vi "Save Recording.vi"(8 "error in":errorcluster, 9 "Save":bool, 11 "Interface In":T1) -> (0 "error out":errorcluster, 1 "Save?":bool, 2 "Data":fxp<+/-,8,8>[](array[numeric]), 3 "Interface Out":T1)   [LabVIEW 2015]
uses:
  TypeDefs Host/FPGA Dynamic Interface.ctl
  TypeDefs Host/Open Audio FGV Enum.ctl
  <vilib>/Utility/error.llb/Error Cluster From Error Code.vi
  <vilib>/rvi/errors/niLvFpgaAdjustHostInterfaceError.vi
  <vilib>/rvi/interface/common/niFpgaWaitOnOcc.vi
  <vilib>/rvi/interface/nirviReadWriteControl/nirviReadWriteControl.xnode
  <vilib>/rvi/interface/nirviMethod/nirviMethod.xnode
  <vilib>/rvi/errors/niLvFpgaMergeErrorWithErrorCode.vi
  <vilib>/FPGAPlugInAG/Dynamic/niLvFpga_ReadFifo_Dynamic.vi
  NiFpgaLv.dll
  <vilib>/rvi/interface/Simulation/niFpgaSimulationCallBeginRW.vi
  <vilib>/FPGAPlugInAG/Dynamic/niLvFpga_ConfigureFifo_Dynamic.vi
  <vilib>/FPGAPlugInAG/Dynamic/niLvFpga_StartFifo_Dynamic.vi
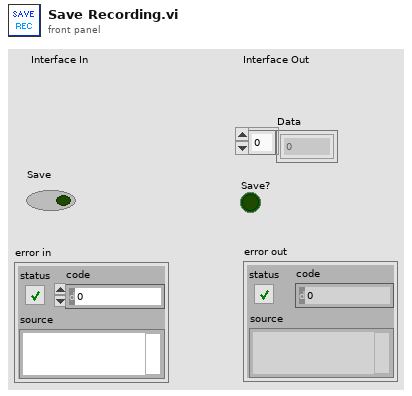
[diagram p1: front panel]
types:
  T1 = typedef "FPGA Dynamic Interface.ctl" = refnum<k20>
  T2 = typedef "Open Audio FGV Enum.ctl" = enum16{"Get", "Set"}
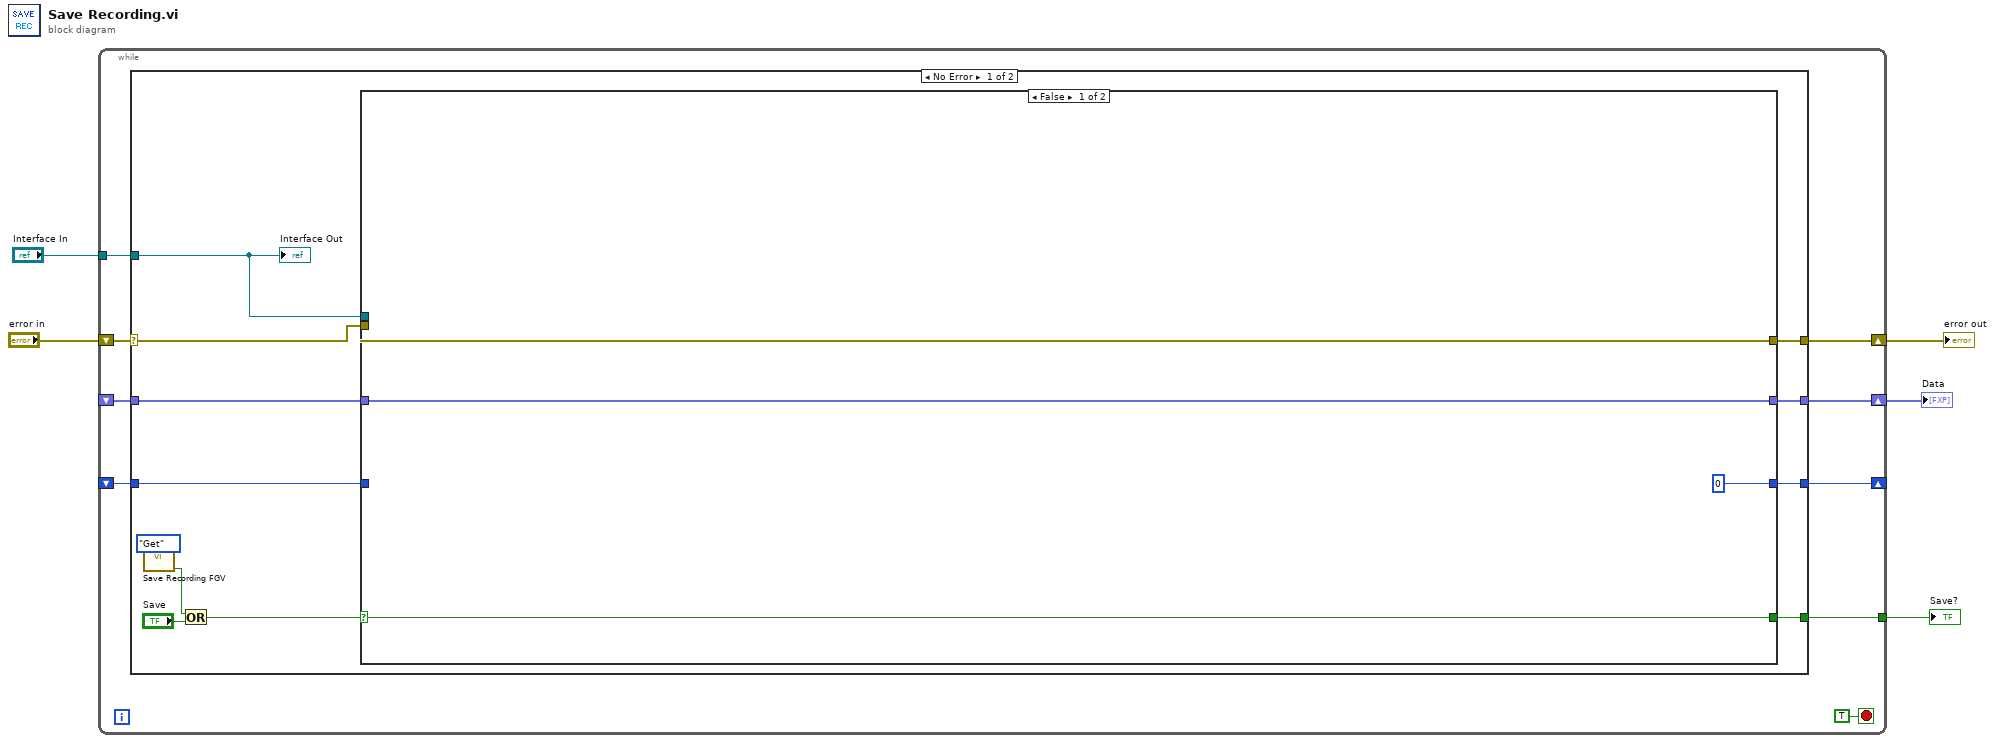
[diagram p0: block diagram]
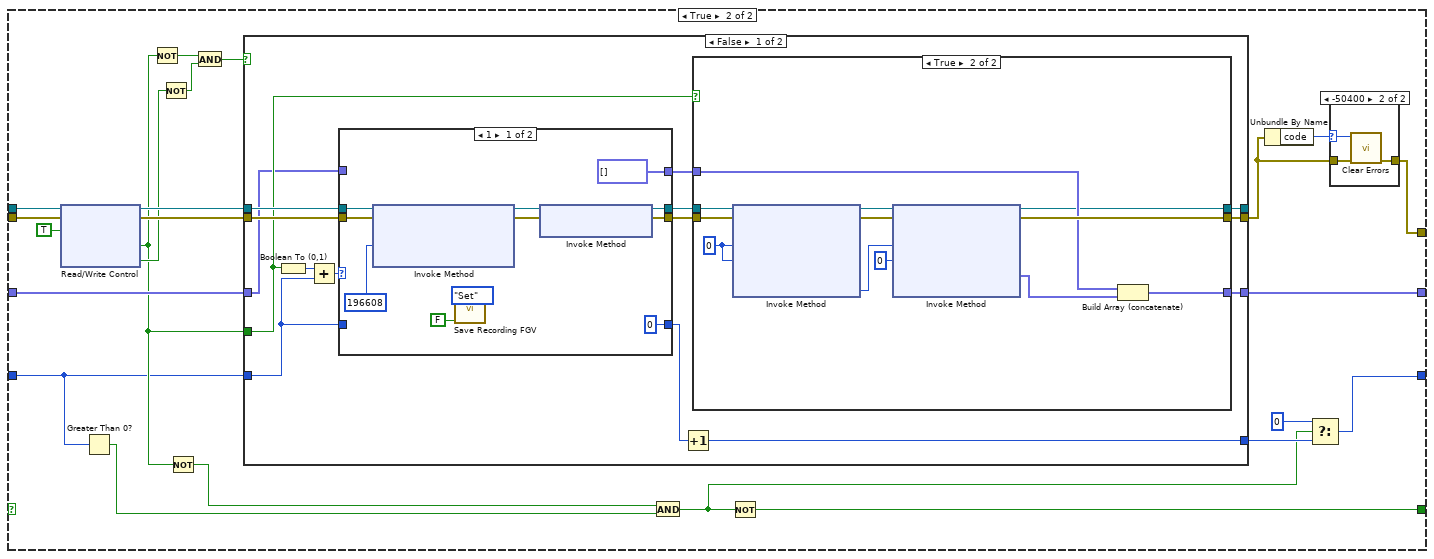
[diagram p2: hidden frame]
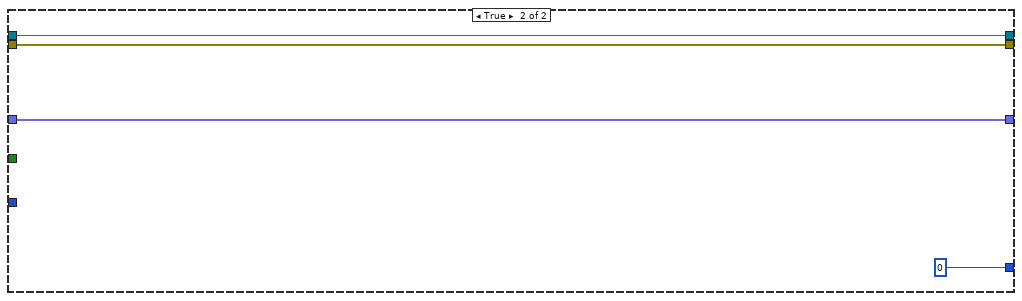
[diagram p6: hidden frame]
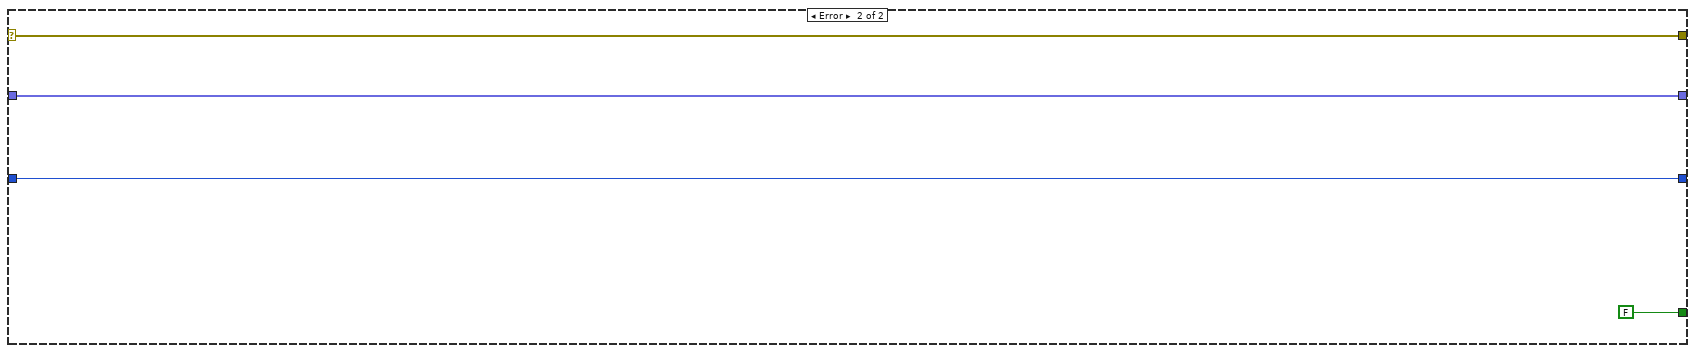
[diagram p7: hidden frame]
diagram:
  n1 = while {
    shift-right: [w10] -> w2
    shift-left: "error in" -> [w7]
    shift-right: [w14] -> w4
    shift-left: _ -> [w12]
    shift-right: [w11] -> _
    shift-left: _ -> [w13]
    tunnel: [w8] -> w3
    tunnel: "Interface In" -> [w6]
    stop <- TRUE stop-if-true
    n2 = case shown="No Error" w7 {
      selector: w7 -> [w16 w110]
      tunnel: [w26 w109] -> w14
      tunnel: w13 -> [w25 w108]
      tunnel: w12 -> [w24 w109]
      tunnel: [w23 w108] -> w11
      tunnel: [w22 w110] -> w10
      tunnel: [w21 FALSE] -> w8
      tunnel: w6 -> [w15 _]
      frame No Error {
        n3 = call "Save Recording FGV.vi"("Command"=Open_Audio_FGV_Enum."Get") -> ("Save?"=w17:bool)  [unwired: 10 in]
        n4 = Or(x=w17, y="Save") -> (x .or. y?=w19:bool)
        n5 = case shown="False" w19 {
          selector: w19 -> [w28 _]
          tunnel: [w29 w53] -> w26
          tunnel: w16 -> [w30 w51]
          tunnel: w25 -> [_ w37]
          tunnel: w24 -> [w29 w47]
          tunnel: [0 ("Chunk size") w40] -> w23
          tunnel: [w30 w41] -> w22
          tunnel: [w28 w34] -> w21
          tunnel: w15 -> [_ w31]
          frame False {
          }
          frame True {
            n6 = xnode "Read/Write Control"("FPGA VI Reference In"=w31, "error in"=w51, "Transfer"=TRUE ("stop")) -> ("FPGA VI Reference Out"=w52:T1, "error out"=w50:errorcluster, "To Host?"=w38:bool, "From Host?"=w39:bool)
            n7 = Greater Than 0?(x=w37) -> (x > 0?=w35:bool)
            n8 = Not(x=w38) -> (.not. x?=w49:bool)
            n9 = Not(x=w39) -> (.not. x?=w48:bool)
            n10 = Not(x=w38) -> (.not. x?=w36:bool)
            n11 = And(x=w49, y=w48) -> (x .and. y?=w44:bool)
            n12 = case shown="False" w44 {
              tunnel: w50 -> [w72 w105]
              tunnel: [w60 w105] -> w42
              tunnel: [w66 w106] -> w53
              tunnel: w47 -> [w61 w106]
              tunnel: w52 -> [w71 w103]
              tunnel: w38 -> [w65 _]
              tunnel: w37 -> [w59 _]
              tunnel: [w62 0 ("Chunk size")] -> w46
              tunnel: [w64 w103] -> _
              frame False {
                n13 = Boolean To (0,1)(Boolean=w65) -> (0, 1=w68:i16)
                n14 = Add(x=w68, y=w59) -> (x+y=w67:i32)
                n15 = case shown="1" w67 {
                  tunnel: w72 -> [w98 w101]
                  tunnel: w71 -> [w97 w102]
                  tunnel: [w94 w102] -> w70
                  tunnel: [w93 w101] -> w69
                  tunnel: w61 -> [_ w100]
                  tunnel: [fxp<+/-,8,8>[] [] ("Data 2") w100] -> w63
                  tunnel: w59 -> [_ w99]
                  tunnel: [0 ("Chunk size") w99] -> w58
                  frame 1 {
                    n16 = xnode "Invoke Method"("FPGA VI Reference In"=w97, "error in"=w98, "Requested Depth"=u32 196608) -> ("FPGA VI Reference Out"=w95:T1, "error out"=w92:errorcluster)  [unwired: 1 out]
                    n17 = call "Save Recording FGV.vi"("Command"=Open_Audio_FGV_Enum."Set", "Save"=FALSE) -> ()  [unwired: 9 in, 1 out]
                    n18 = xnode "Invoke Method"("FPGA VI Reference In"=w95, "error in"=w92) -> ("FPGA VI Reference Out"=w94:T1, "error out"=w93:errorcluster)
                  }
                  frame 0, Default {
                  }
                }
                n19 = Increment(x=w58) -> (x+1=w62:i32)
                n20 = case shown="True" w65 {
                  tunnel: [w74 w87] -> w60
                  tunnel: [w75 w77] -> w64
                  tunnel: w70 -> [w75 w85]
                  tunnel: w69 -> [w74 w79]
                  tunnel: [w73 w82] -> w66
                  tunnel: w63 -> [w73 w81]
                  frame False {
                  }
                  frame True {
                    w76 = u32 0 ("Number of Elements")
                    n21 = xnode "Invoke Method"("FPGA VI Reference In"=w85, "error in"=w79, "Number of Elements"=w76, "Timeout (ms)"=w76) -> ("FPGA VI Reference Out"=w84:T1, "error out"=w78:errorcluster, "Elements Remaining"=w80:u32)  [unwired: 1 out]
                    n22 = xnode "Invoke Method"("FPGA VI Reference In"=w84, "error in"=w78, "Number of Elements"=w80, "Timeout (ms)"=0) -> ("FPGA VI Reference Out"=w77:T1, "error out"=w87:errorcluster, "Data"=w83:fxp<+/-,8,8>[])  [unwired: 1 out]
                    n23 = Build Array (concatenate)(w81, w83) -> (w82:fxp<+/-,8,8>[])
                  }
                }
              }
              frame True {
              }
            }
            n24 = And(x=w36, y=w35) -> (x .and. y?=w33:bool)
            n25 = Not(x=w33) -> (.not. x?=w34:bool)
            n26 = Unbundle By Name(w42) -> ("code"=w43:i32)
            n27 = Select(t=0, s=w33, f=w46) -> (s? t:f=w40:i32)
            n28 = case shown="-50400" w43 {
              selector: w43 -> [_ w57]
              tunnel: w42 -> [w54 w56]
              tunnel: [w54 w55] -> w41
              frame 0, Default {
              }
              frame -50400 {
                n29 = call <vilib>:"Clear Errors.vi"("error in (no error)"=w56, "specific error code to clear (0: all)"=w57) -> ("error out"=w55:errorcluster)  [unwired: 4 in, 1 out]
              }
            }
          }
        }
        "Interface Out" <- w15
      }
      frame Error {
      }
    }
  }
  "error out" <- w2
  "Data" <- w4
  "Save?" <- w3
